vi "Handle PUBLISHED.vi"(8 "error in (no error)":errorcluster, 9 "Message Loop data (in)":T1, 10 "WAMP Message":T16 {"Message Codes" items=["HELLO"=1, "WELCOME"=2, "ABORT"=3, "GOODBYE"=6, "ERROR"=8, "PUBLISH"=16, "PUBLISHED"=17, "SUBSCRIBE"=32, "SUBSCRIBED"=33, "UNSUBSCRIBE"=34, "UNSUBSCRIBED"=35, "EVENT"=36, "CALL"=48, "RESULT"=59, "REGISTER"=64, "REGISTERED"=65, "UNREGISTER"=66, "UNREGISTERED"=67, "INVOCATION"=68, "YIELD"=70]}, 11 "reference":refnum<class "WAMP Client.lvclass">) -> (0 "error out":errorcluster, 1 "Message Loop data (out)":T1, 3 "reference out":refnum<class "WAMP Client.lvclass">)   [LabVIEW 2020, in "wamplv.lvlib" / "WAMP Client.lvclass"]
uses:
  WAMP Client.lvclass
  TypeDef/WAMP Received Message.ctl
  TypeDef/WAMP Message Codes.ctl
  TypeDef/Message Loop Data.ctl
  TypeDef/REGISTER Request Data.ctl
  TypeDef/Success or error.ctl
  API/TypeDefs/Combined error.ctl
  API/TypeDefs/WAMP error.ctl
  TypeDef/Publish Requests Map.ctl
  TypeDef/PUBLISH Request Data.ctl
  TypeDef/PUBLISH result.ctl
  TypeDef/Endpoint Data.ctl
  TypeDef/CALL Request Map.ctl
  TypeDef/CALL request (JSON).ctl
  API/TypeDefs/RESULT payload (JSON).ctl
  TypeDef/SUBSCRIBE Requests Map.ctl
  TypeDef/SUBSCRIBE Request Data.ctl
  TypeDef/Subscribe Result.ctl
  TypeDef/EVENT payload.ctl
  TypeDef/Subscriptions Map.ctl
  TypeDef/Subscription Details.ctl
  TypeDef/Unsubscribe Requests Map.ctl
  TypeDef/UNSUBSCRIBE Request Data.ctl
  TypeDef/UNSUBSCRIBE Result.ctl
  TypeDef/Unregister requests map.ctl
  TypeDef/Unregister request.ctl
  e5b7c8eb-71f6-44ee-8f98-5a3218503335.vi
  WAMP Client.lvclass/WAMP Client.ctl
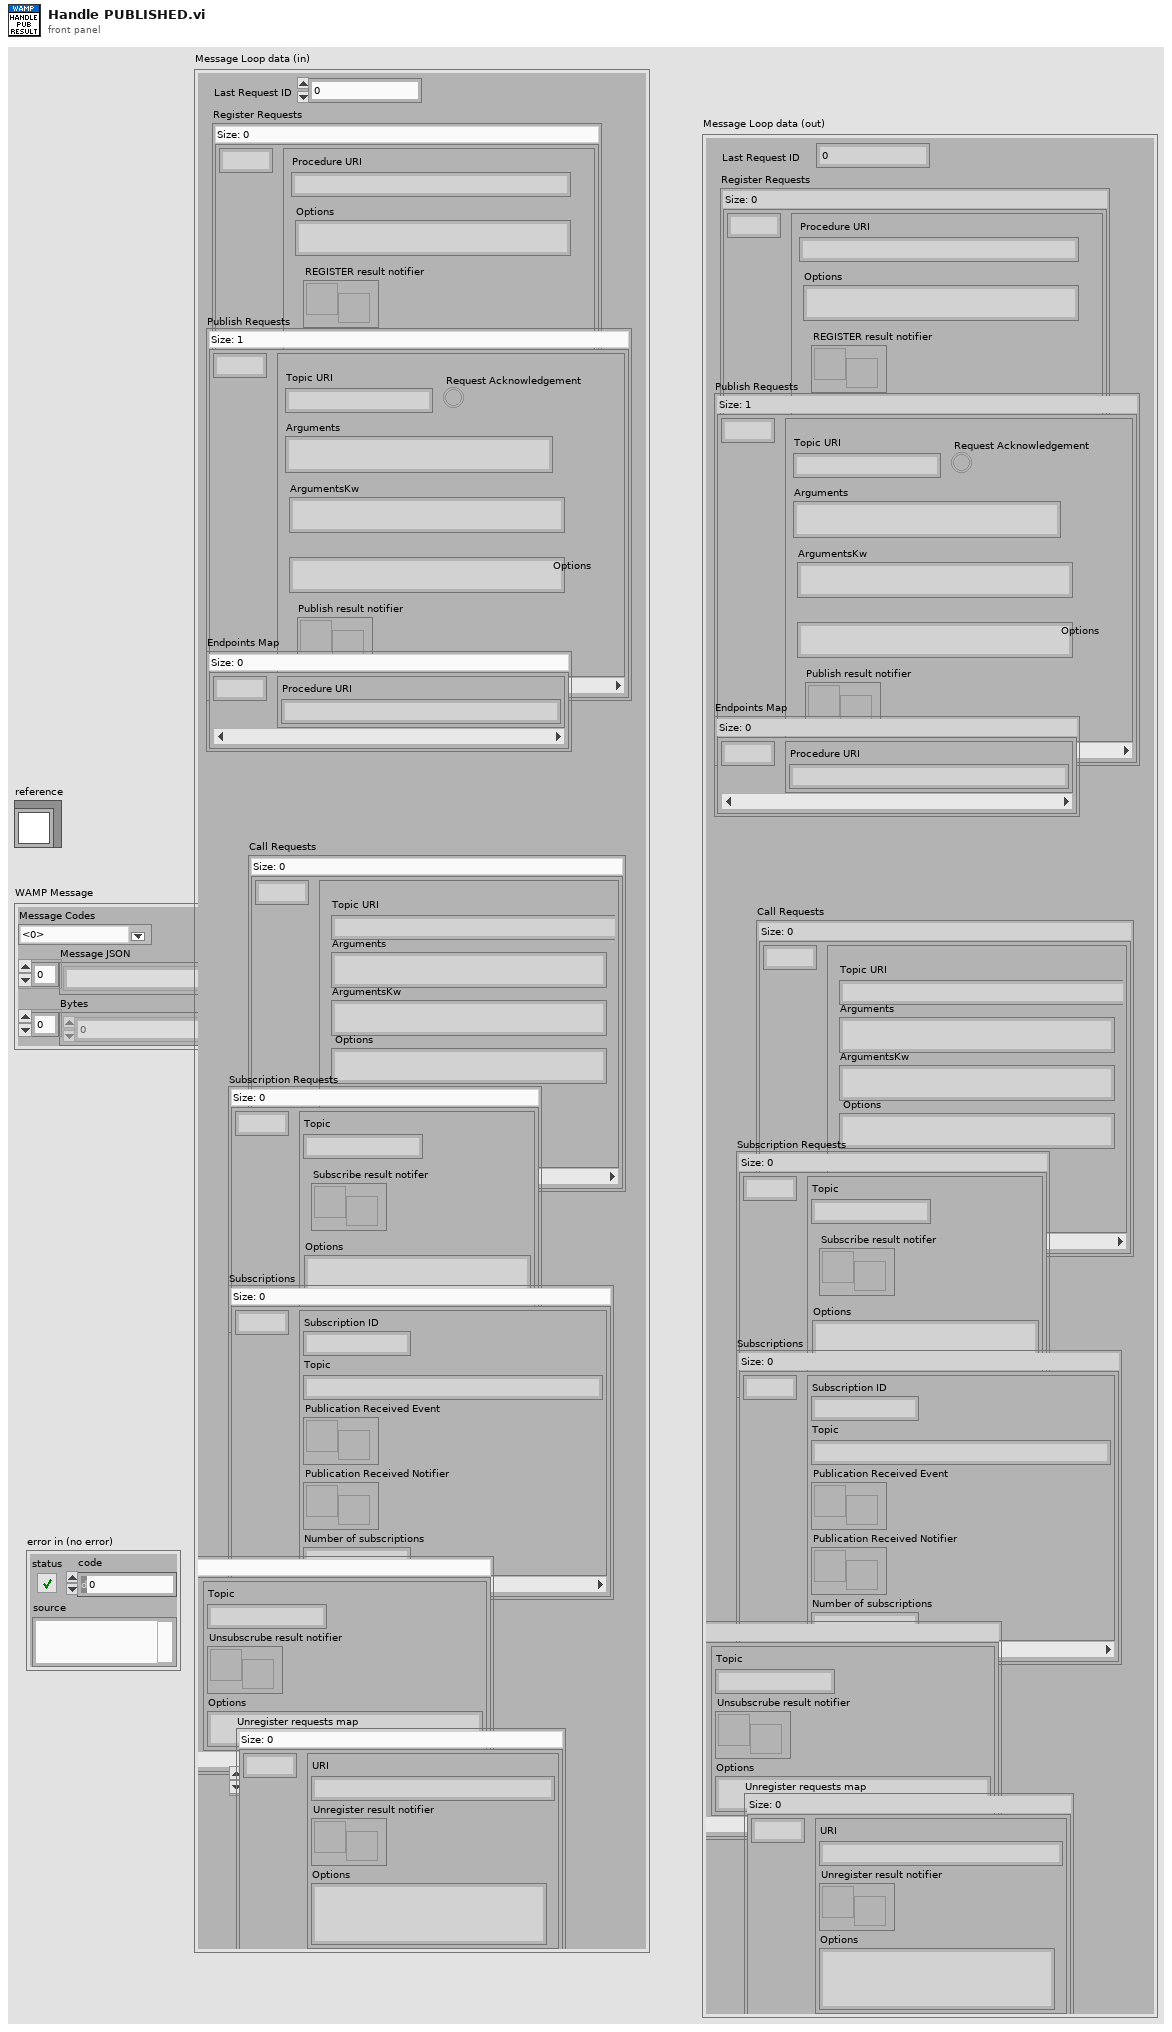
[diagram p1: front panel]
types:
  T1 = typedef "wamplv.lvlib/WAMP Client.lvclass/Message Loop Data.ctl" = cluster{"Last Request ID":u64, "Register Requests":map{u64, T2}, "Publish Requests":T3, "Endpoints Map":map{u64, T5}, "Call Requests":T6, "Subscription Requests":T8, "Subscriptions":T10, "Unsubscribe Requests":T12, "Random Request IDs":u64[], "Unregister requests map":T14}
  T2 = typedef "wamplv.lvlib/WAMP Client.lvclass/REGISTER Request Data.ctl" = cluster{"Procedure URI":string, "Options":string, "REGISTER result notifier":refnum<notifier>}
  T3 = typedef "wamplv.lvlib/WAMP Client.lvclass/Publish Requests Map.ctl" = map{u64, T4}
  T4 = typedef "wamplv.lvlib/WAMP Client.lvclass/PUBLISH Request Data.ctl" = cluster{"Topic URI":string, "Arguments":string, "ArgumentsKw":string, "Request Acknowledgement":bool, "Options":string, "Publish result notifier":refnum<notifier>}
  T5 = typedef "wamplv.lvlib/WAMP Client.lvclass/Endpoint Data.ctl" = cluster{"Procedure URI":string}
  T6 = typedef "wamplv.lvlib/WAMP Client.lvclass/CALL Request Map.ctl" = map{u64, T7}
  T7 = typedef "wamplv.lvlib/WAMP Client.lvclass/CALL request (JSON).ctl" = cluster{"Topic URI":string, "Arguments":string, "ArgumentsKw":string, "Options":string, "Call result":refnum<notifier>}
  T8 = typedef "wamplv.lvlib/WAMP Client.lvclass/SUBSCRIBE Requests Map.ctl" = map{u64, T9}
  T9 = typedef "wamplv.lvlib/WAMP Client.lvclass/SUBSCRIBE Request Data.ctl" = cluster{"Topic":string, "Subscribe result notifer":refnum<notifier>, "Options":string}
  T10 = typedef "wamplv.lvlib/WAMP Client.lvclass/Subscriptions Map.ctl" = map{u64, T11}
  T11 = typedef "wamplv.lvlib/WAMP Client.lvclass/Subscription Details.ctl" = cluster{"Subscription ID":u64, "Topic":string, "Publication Received Event":refnum<user-event>, "Publication Received Notifier":refnum<notifier>, "Number of subscriptions":u64}
  T12 = typedef "wamplv.lvlib/WAMP Client.lvclass/Unsubscribe Requests Map.ctl" = map{u64, T13}
  T13 = typedef "wamplv.lvlib/WAMP Client.lvclass/UNSUBSCRIBE Request Data.ctl" = cluster{"Topic":string, "Unsubscrube result notifier":refnum<notifier>, "Options":string}
  T14 = typedef "wamplv.lvlib/WAMP Client.lvclass/Unregister requests map.ctl" = map{u64, T15}
  T15 = typedef "wamplv.lvlib/WAMP Client.lvclass/Unregister request.ctl" = cluster{"URI":string, "Unregister result notifier":refnum<notifier>, "Options":string}
  T16 = typedef "wamplv.lvlib/WAMP Client.lvclass/WAMP Received Message.ctl" = cluster{"Message Codes":T17, "Message JSON":string[], "Bytes":u8[]}
  T17 = typedef "wamplv.lvlib/WAMP Client.lvclass/WAMP Message Codes.ctl" = u16
  T18 = typedef "wamplv.lvlib/WAMP Client.lvclass/PUBLISH result.ctl" = cluster{"Publication ID":u64, "Success?":bool, "Combined Error":T19}
  T19 = typedef "wamplv.lvlib/WAMP Client.lvclass/Combined error.ctl" = cluster{"Error?":bool, "WAMP Error":T20, "Error":errorcluster}
  T20 = typedef "wamplv.lvlib/WAMP Client.lvclass/WAMP error.ctl" = cluster{"Details":string, "ArgumentKw Payload":string, "Error?":bool, "Error URI":string, "Arguments Payload":string}
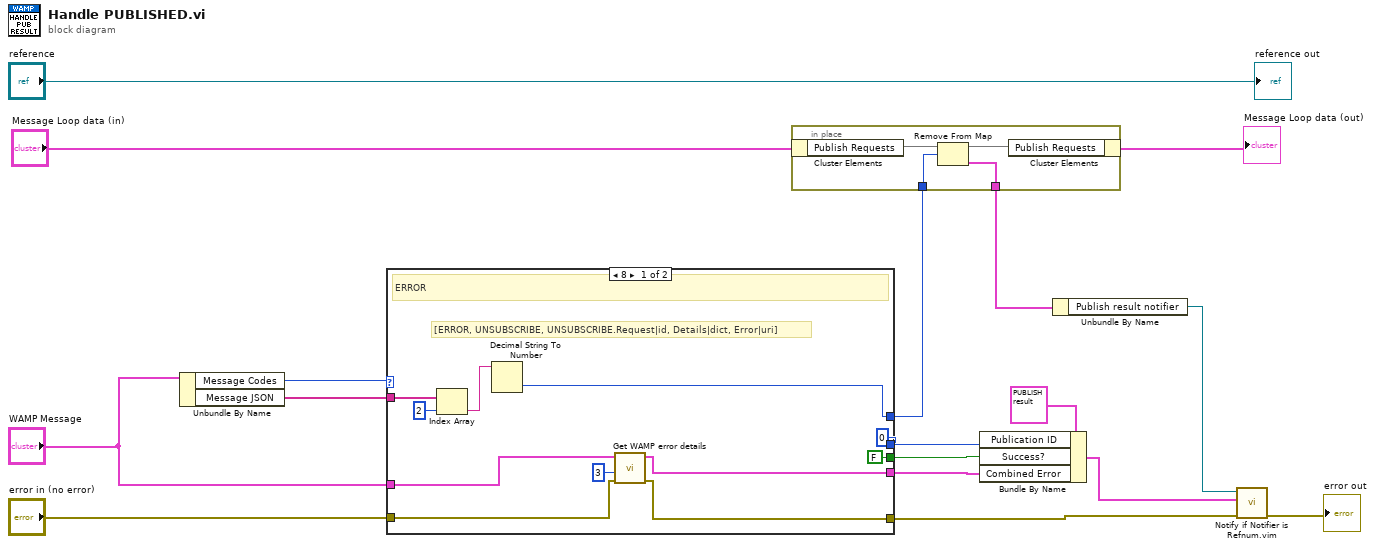
[diagram p0: block diagram]
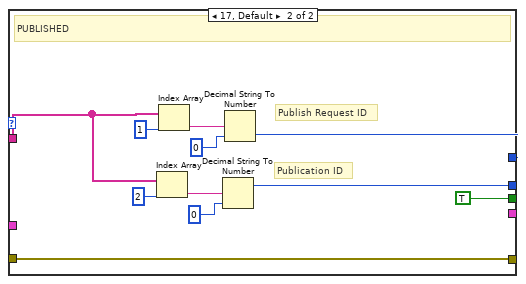
[diagram p2: hidden frame]
diagram:
  n1 = Unbundle By Name("WAMP Message") -> ("Message Codes"=w14:T17, "Message JSON"=w13:string[])
  n2 = case shown="8" w14 {
    tunnel: w13 -> [w26 w30]
    tunnel: [w24 w34] -> w10
    tunnel: "error in (no error)" -> [w18 w38]
    tunnel: [w19 w38] -> w4
    tunnel: [FALSE ("Success?") TRUE ("Success?")] -> w16
    tunnel: [0 ("offset past number") w29] -> w9
    tunnel: "WAMP Message" -> [w22 _]
    tunnel: [w20 _] -> w7
    frame 8 {
      # "[ERROR, UNSUBSCRIBE, UNSUBSCRIBE.Request|id, Details|dict, Error|uri]"
      # "ERROR"
      n3 = Index Array(array=w26, index=2) -> (element=w27:string)
      n4 = Decimal String To Number(string=w27) -> (number=w24:i32)  [unwired: 2 in, 1 out]
      n5 = call "Get WAMP error details.vi"("error in (no error)"=w18, "Details Index"=u32 3, "WAMP Message"=w22) -> ("error out"=w19:errorcluster, "Combined Error"=w20:T19)  [unwired: 6 in, 1 out]
    }
    frame 17, Default {
      # "Publication ID"
      # "Publish Request ID"
      # "PUBLISHED"
      n6 = Index Array(array=w30, index=2) -> (element=w32:string)
      n7 = Index Array(array=w30, index=1) -> (element=w36:string)
      n8 = Decimal String To Number(string=w32, default (0L)=u64 0) -> (offset past number=w29:i32)  [unwired: 1 in, 1 out]
      n9 = Decimal String To Number(string=w36, default (0L)=u64 0) -> (number=w34:u64)  [unwired: 1 in, 1 out]
    }
  }
  n10 = in-place "In Place Element Structure" {
    in-place-border: [w43] -> w12
    in-place-border: w10 -> [w42]
    n11 = in-place-cluster #1("Message Loop data (in)") -> ("Publish Requests"=w41:T3)
    n12 = Remove From Map(10:w42, 11:w41) -> (1:w43:T4, 3:w40:T3)  [unwired: 1 out]
    n13 = in-place-cluster #1("Publish Requests"=w40) -> (→"Message Loop data (out)":T1)
  }
  n14 = Bundle By Name(cluster=T18 {"Publication ID"=0, "Success?"=FALSE, "Combined Error"={"Error?"=FALSE, "WAMP Error"={"Details"="", "ArgumentKw Payload"="{}", "Error?"=FALSE, "Error URI"="", "Arguments Payload"=""}, "Error"={"status"=FALSE, "code"=0, "source"=""}}} ("Cluster"), "Publication ID"=w9, "Success?"=w16, "Combined Error"=w7) -> (w5:T18)
  n15 = Unbundle By Name(w12) -> ("Publish result notifier"=w6:refnum<notifier>)
  n16 = call "Notify if Notifier is Refnum.vim"("error in (no error)"=w4, "RESULT Payload"=w5, "Notifier in"=w6) -> ("error out"=→"error out":errorcluster)  [unwired: 8 in]
  "reference out" <- "reference"
